vi "Connection_Arduino.vi"(0 "VISA resource name":refnum<visa-resource-name>, 1 "baud rate (9600)":u32=9600) -> (2 "VISA resource name out":refnum<visa-resource-name>, 3 "Slide":u8(slide) scale=0.0..100.0, 4 "error out":errorcluster, 5 "Boolean":bool)   [LabVIEW 2018]
uses:
  <vilib>/Instr/_visa.llb/VISA Configure Serial Port (Instr).vi
panel:
  out "Out":string
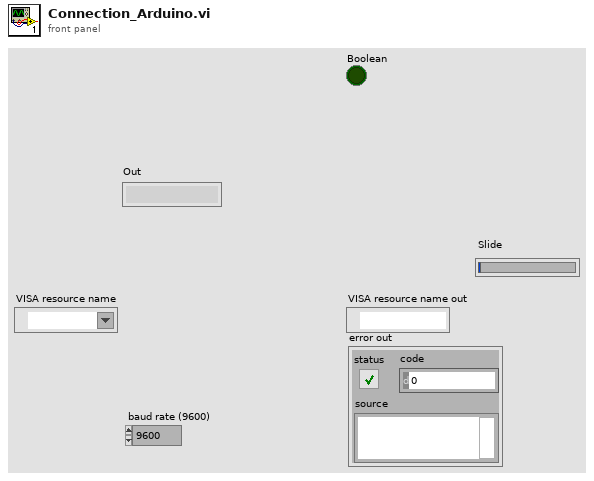
[diagram p1: front panel]
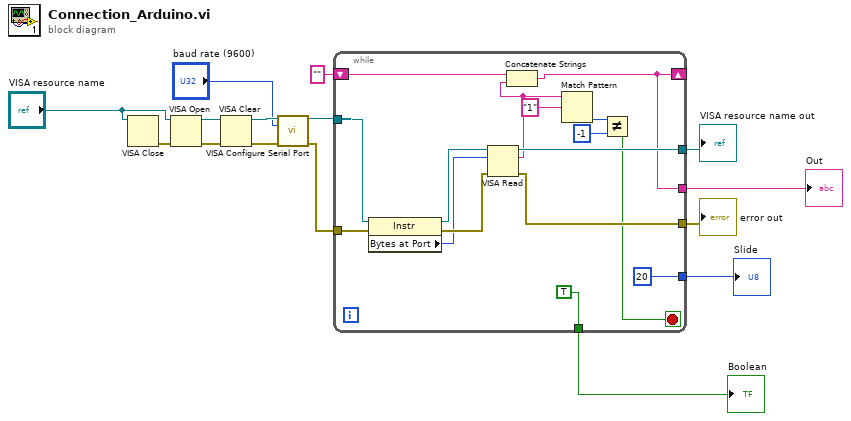
[diagram p0: block diagram]
diagram:
  n1 = VISA Close(VISA resource name="VISA resource name") -> (error out=w15:errorcluster)  [unwired: 1 in]
  n2 = VISA Open(error in (no error)=w15, VISA resource name="VISA resource name") -> (VISA resource name=w14:refnum<visa-resource-name>, error out=w13:errorcluster)  [unwired: 3 in]
  n3 = VISA Clear(VISA resource name=w14, error in (no error)=w13) -> (VISA resource name out=w11:refnum<visa-resource-name>, error out=w10:errorcluster)
  n4 = call-poly "VISA Configure Serial Port"("VISA resource name"=w11, "baud rate (9600)"="baud rate (9600)", "error in (no error)"=w10) -> ("VISA resource name out"=w8:refnum<visa-resource-name>, "error out"=w7:errorcluster)  [unwired: 11 in]
  n5 = while {
    tunnel: w8 -> [w31]
    tunnel: w7 -> [w30]
    tunnel: [w26] -> w6
    tunnel: [w25] -> w5
    shift-right: [w18] -> _
    shift-left: "" -> [w21]
    tunnel: [w18] -> w4
    tunnel: [u8 20 ("Slide")] -> w2
    tunnel: [TRUE ("Boolean")] -> w1
    stop <- w19 stop-if-true
    n6 = property class="Instr"(reference=w31, error in=w30) -> (reference out=w29:refnum<visa-resource-name>, error out=w28:errorcluster, "Bytes at Port"=w27:u32)
    n7 = VISA Read(VISA resource name=w29, byte count=w27, error in (no error)=w28) -> (VISA resource name out=w26:refnum<visa-resource-name>, read buffer=w23:string, error out=w25:errorcluster)  [unwired: 1 out]
    n8 = Concatenate Strings(w21, w23) -> (w18:string)
    n9 = Match Pattern(string=w23, regular expression="1") -> (offset past match=w24:i32)  [unwired: 1 in, 3 out]
    n10 = Not Equal?(x=w24, y=-1) -> (x != y?=w19:bool)
  }
  "VISA resource name out" <- w6
  "error out" <- w5
  "Out" <- w4
  "Slide" <- w2
  "Boolean" <- w1
